vi "LV Image to Jpeg string.vi"() -> ()   [LabVIEW 2016]
uses:
  System.Drawing
panel:
  in  "JPEG File":path
  out "Jpeg String":string
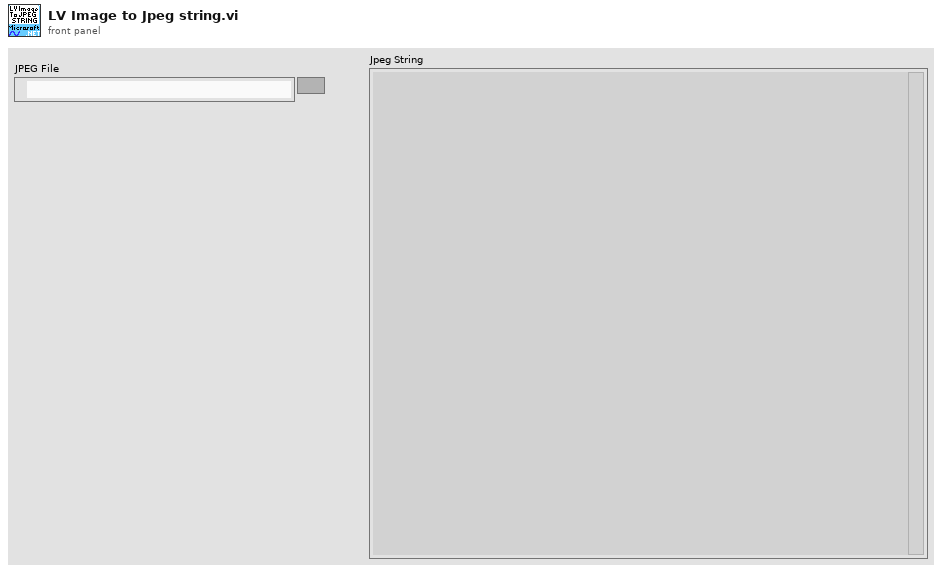
[diagram p1: front panel]
types:
  T1 = typedef "imagedata.ctl" = cluster{"image type":i32, "image depth":i32, "image":u8[], "mask":u8[], "colors":u32[], "Rectangle":cluster{"left":i16, "top":i16, "right":i16, "bottom":i16}}
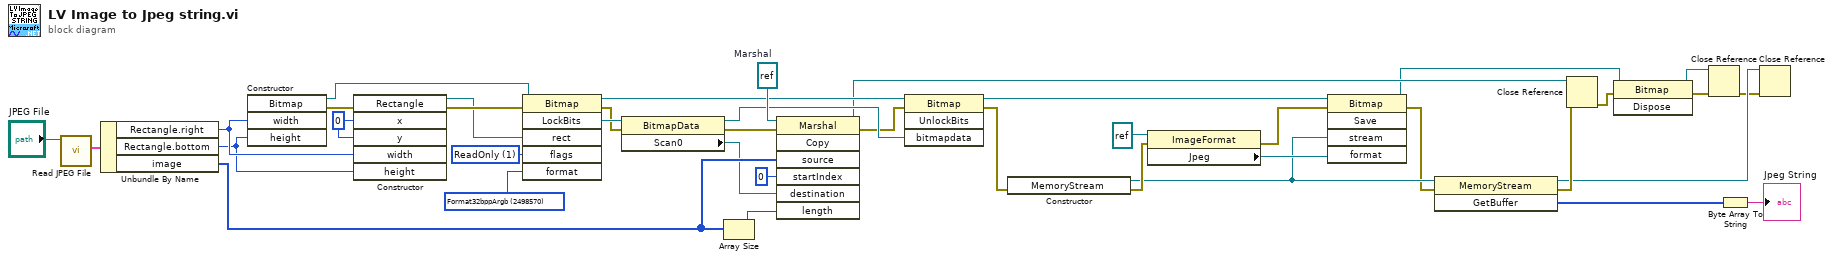
[diagram p0: block diagram]
diagram:
  w19 = refnum<k24> refnum  # Marshal
  w22 = 2498570 items=["DontCare, Undefined"=0, "Max"=15, "Indexed"=65536, "Gdi"=131072, "Format16bppRgb555"=135173, "Format16bppRgb565"=135174, "Format24bppRgb"=137224, "Format32bppRgb"=139273, "Format1bppIndexed"=196865, "Format4bppIndexed"=197634, "Format8bppIndexed"=198659, "Alpha"=262144, "Format16bppArgb1555"=397319, "PAlpha"=524288, "Format32bppPArgb"=925707, "Extended"=1048576, "Format16bppGrayScale"=1052676, "Format48bppRgb"=1060876, "Format64bppPArgb"=1851406, "Canonical"=2097152, "Format32bppArgb"=2498570, "Format64bppArgb"=3424269] ("format")
  w23 = 1 items=["ReadOnly"=1, "WriteOnly"=2, "ReadWrite"=3, "UserInputBuffer"=4] ("flags")
  w30 = 0 ("x")
  n1 = call <vilib>:"Read JPEG File.vi"("path to JPEG file"="JPEG File") -> ("image data"=w37:T1)  [unwired: 8 in, 2 out]
  n2 = Unbundle By Name(w37) -> ("Rectangle.right"=w29:i16, "Rectangle.bottom"=w28:i16, "image"=w16:u8[])
  n3 = constructor class="Bitmap"("width"=w29, "height"=w28) -> (reference out=w26:refnum<k24>, error out=w27:errorcluster)  [unwired: 3 in, 3 out]
  n4 = constructor class="Rectangle"(error in=w27, "x"=w30, "y"=w30, "width"=w29, "height"=w28) -> (reference out=w24:refnum<k24>, error out=w25:errorcluster)  [unwired: 2 in, 5 out]
  n5 = invoke class="Bitmap" method="LockBits"(reference=w26, error in=w25, "rect"=w24, "flags"=w23, "format"=w22) -> (reference out=w13:refnum<k24>, error out=w20:errorcluster, "LockBits"=w21:refnum<k24>)  [unwired: 1 in, 3 out]
  n6 = property class="BitmapData"(reference=w21, error in=w20) -> (reference out=w12:refnum<k24>, error out=w18:errorcluster, "Scan0"=w15:refnum<k24>)
  n7 = Array Size(array=w16) -> (size(s)=w14:i32)
  n8 = invoke class="Marshal" method="Copy"(reference=w19, error in=w18, "source"=w16, "startIndex"=0, "destination"=w15, "length"=w14) -> (reference out=w7:refnum<k24>, error out=w11:errorcluster)  [unwired: 1 in, 5 out]
  n9 = invoke class="Bitmap" method="UnlockBits"(reference=w13, error in=w11, "bitmapdata"=w12) -> (reference out=w10:refnum<k24>, error out=w9:errorcluster)  [unwired: 1 in, 2 out]
  n10 = constructor class="MemoryStream"(error in=w9) -> (reference out=w32:refnum<k24>, error out=w34:errorcluster)  [unwired: 2 in, 1 out]
  n11 = property class="ImageFormat"(reference=refnum<k24> refnum ("format"), error in=w34) -> (error out=w33:errorcluster, "Jpeg"=w35:refnum<k24>)  [unwired: 1 out]
  n12 = invoke class="Bitmap" method="Save"(reference=w10, error in=w33, "stream"=w32, "format"=w35) -> (reference out=w6:refnum<k24>, error out=w31:errorcluster)  [unwired: 1 in, 3 out]
  n13 = invoke class="MemoryStream" method="GetBuffer"(reference=w32, error in=w31) -> (reference out=w2:refnum<k24>, error out=w8:errorcluster, "GetBuffer"=w40:u8[])  [unwired: 1 in]
  n14 = Close Reference(reference=w7, error in (no error)=w8) -> (error out=w5:errorcluster)
  n15 = invoke class="Bitmap" method="Dispose"(reference=w6, error in=w5) -> (reference out=w3:refnum<k24>, error out=w4:errorcluster)  [unwired: 1 in, 1 out]
  n16 = Close Reference(reference=w3, error in (no error)=w4) -> (error out=w1:errorcluster)
  n17 = Byte Array To String(unsigned byte array=w40) -> (string=→"Jpeg String":string)
  n18 = Close Reference(reference=w2, error in (no error)=w1) -> ()  [unwired: 1 out]
